vi "Get Channel Model Number.vi"(8 "error in (no error)":errorcluster {"code" format="%.0x"}, 10 "Channel Name (1)":string="1", 11 "VISA resource name":refnum<visa-resource-name>) -> (0 "error out":errorcluster {"code" format="%.0x"}, 2 "Model Number":string, 3 "VISA resource name out":refnum<visa-resource-name>)   [LabVIEW 2014, in "Agilent N6700 Series.lvlib"]
doc: "Returns model number for the channel name entered."
uses:
  Agilent N6700 Series.lvlib
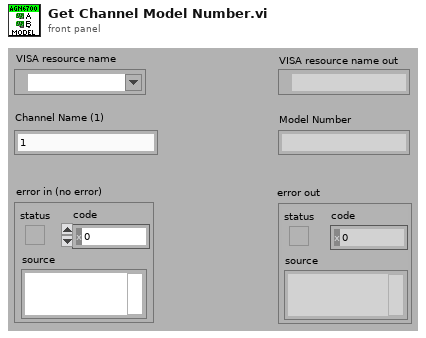
[diagram p1: front panel]
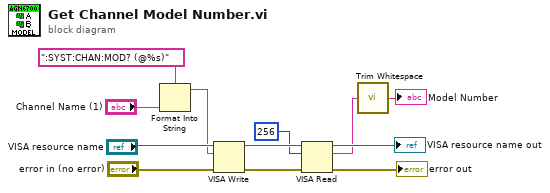
[diagram p0: block diagram]
diagram:
  n1 = Format Into String(format string=":SYST:CHAN:MOD? (@%s)", "Channel Name (1)") -> (resulting string=w3:string)  [unwired: 2 in, 1 out]
  n2 = VISA Write(VISA resource name="VISA resource name", write buffer=w3, error in (no error)="error in (no error)") -> (VISA resource name out=w10:refnum<visa-resource-name>, error out=w9:errorcluster)  [unwired: 1 out]
  n3 = VISA Read(VISA resource name=w10, byte count=u32 256, error in (no error)=w9) -> (VISA resource name out=→"VISA resource name out":refnum<visa-resource-name>, read buffer=w1:string, error out=→"error out":errorcluster)  [unwired: 1 out]
  n4 = call "Trim Whitespace.vi"("string"=w1) -> ("trimmed string"=→"Model Number":string)  [unwired: 1 in]
